vi "Normalize with Lowest Den Term (DBL).vi"(10 "Denominator":dbl[](array[numeric]), 11 "Numerator":dbl[](array[numeric])) -> (0 "error":i32, 2 "Normalized Denominator":dbl[](array[numeric]), 3 "Normalized Numerator":dbl[](array[numeric]))   [LabVIEW 2020, in "NI_AALPro.lvlib"]
doc: "Normalizes numerator and denominator polynomials with the lowest denominator term. The data types you wire to the <B>Numerator</B> and <B>Denominator</B> inputs determine the polymorphic instance to use."
uses:
  NI_AALPro.lvlib
  Remove Zero Coefficients (DBL).vi
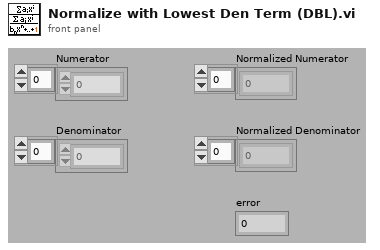
[diagram p1: front panel]
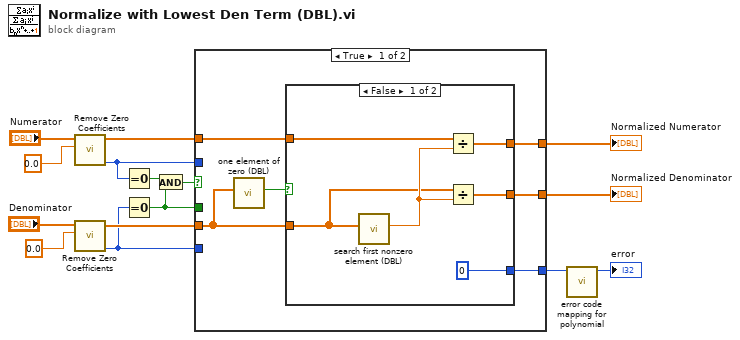
[diagram p0: block diagram]
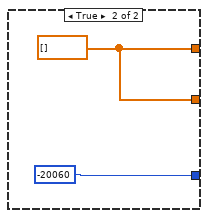
[diagram p2: hidden frame]
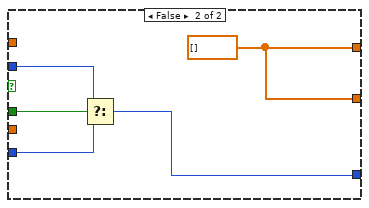
[diagram p3: hidden frame]
diagram:
  n1 = call-poly "Remove Zero Coefficients.vi"("threshold"=0.0, "P(x) In"="Numerator") -> ("error"=w5:i32, "P(x) Out"=w9:dbl[])  [unwired: 7 in, 1 out]
  n2 = call-poly "Remove Zero Coefficients.vi"("threshold"=0.0, "P(x) In"="Denominator") -> ("error"=w4:i32, "P(x) Out"=w11:dbl[])  [unwired: 7 in, 1 out]
  n3 = Equal To 0?(x=w5) -> (x = 0?=w2:bool)
  n4 = Equal To 0?(x=w4) -> (x = 0?=w1:bool)
  n5 = And(x=w2, y=w1) -> (x .and. y?=w3:bool)
  n6 = case shown="True" w3 {
    tunnel: [w21 w34] -> w15
    tunnel: [w20 w34] -> w14
    tunnel: w11 -> [w18 _]
    tunnel: w9 -> [w19 _]
    tunnel: [w16 w31] -> w7
    tunnel: w5 -> [_ w33]
    tunnel: w4 -> [_ w32]
    tunnel: w1 -> [_ w30]
    frame True {
      n7 = call "one element of zero (DBL).vi"("Array in"=w18) -> ("equal [0]?"=w17:bool)  [unwired: 10 in]
      n8 = case shown="False" w17 {
        tunnel: [w27 w29] -> w21
        tunnel: [w26 w29] -> w20
        tunnel: w18 -> [w22 _]
        tunnel: w19 -> [w25 _]
        tunnel: [0 -20060 ("divide by zero")] -> w16
        frame False {
          n9 = call "search first nonzero element (DBL).vi"("Numbers"=w22) -> ("first nonzero element"=w23:dbl)  [unwired: 10 in]
          n10 = Divide(x=w25, y=w23) -> (x/y=w26:dbl[])
          n11 = Divide(x=w22, y=w23) -> (x/y=w27:dbl[])
        }
        frame True {
          w29 = dbl[] [] ("BDL")
        }
      }
    }
    frame False {
      w34 = dbl[] [] ("BDL")
      n12 = Select(t=w33, s=w30, f=w32) -> (s? t:f=w31:i32)
    }
  }
  "Normalized Denominator" <- w15
  "Normalized Numerator" <- w14
  n13 = call "error code mapping for polynomial.vi"("error in"=w7) -> ("error out"=→"error":i32)  [unwired: 10 in]
